vi "Validate Range.vi"(8 "error in (no error)":errorcluster, 10 "Range":T1, 11 "Scanner in":refnum<class "Scanner.lvclass">) -> (0 "error out":errorcluster, 2 "Validated Range":T1, 3 "Scanner out":refnum<class "Scanner.lvclass">)   [LabVIEW 2023, in "Scanner.lvclass"]
doc: "Coerce the range to be within this Scanner's physical limits."
uses:
  Scanner.lvclass
  Range.ctl
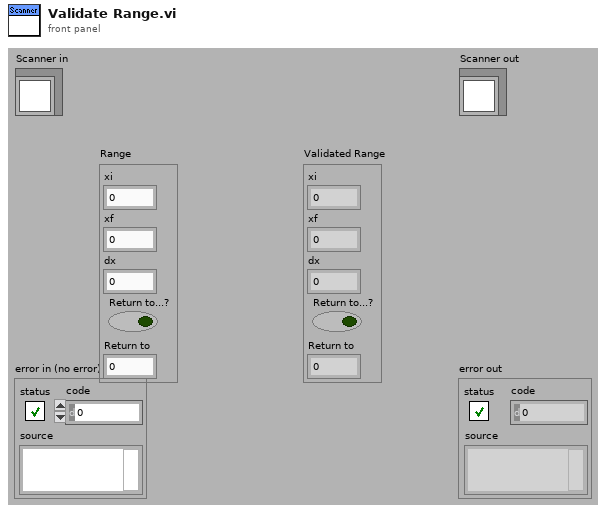
[diagram p1: front panel]
types:
  T1 = typedef "Scanner.lvclass/Range.ctl" = cluster{"xi":dbl, "xf":dbl, "dx":dbl, "Return to...?":bool, "Return to":dbl}
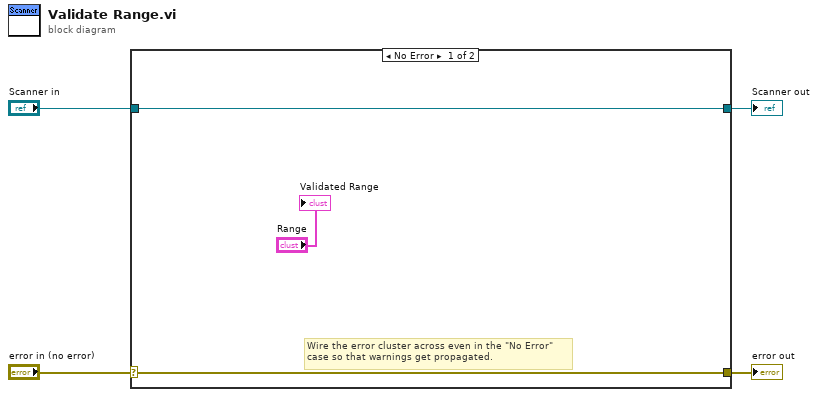
[diagram p0: block diagram]
diagram:
  n1 = case shown="No Error" "error in (no error)" {
    selector: "error in (no error)" -> [w6 w9]
    tunnel: [w6 w9] -> w3
    tunnel: [w7 w8] -> w1
    tunnel: "Scanner in" -> [w7 w8]
    frame No Error {
      # "Wire the error cluster across even in the \"No Error\"\ncase so that warnings get propagated."
      "Validated Range" <- "Range"
    }
    frame Error {
    }
  }
  "error out" <- w3
  "Scanner out" <- w1
